vi "WriteBit.vi"(8 "Error In":errorcluster, 9 "State":bool, 10 "Line (1-14)":u8=1 min=1 max=14 step=1, 11 "Keithley 2602 In":refnum<visa-resource-name>) -> (0 "Error Out":errorcluster, 3 "Keithley 2602 Out":refnum<visa-resource-name>)   [LabVIEW 2012, in "Keithley-2602.lvlib"]
uses:
  Keithley-2602.lvlib
panel:
  out "concatenated string":string
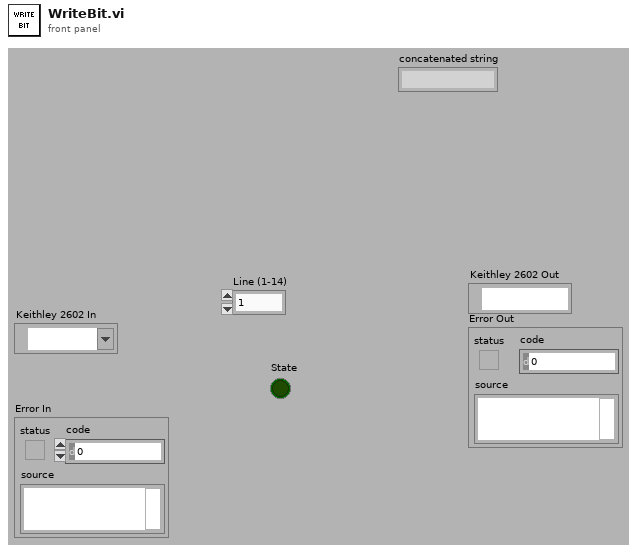
[diagram p1: front panel]
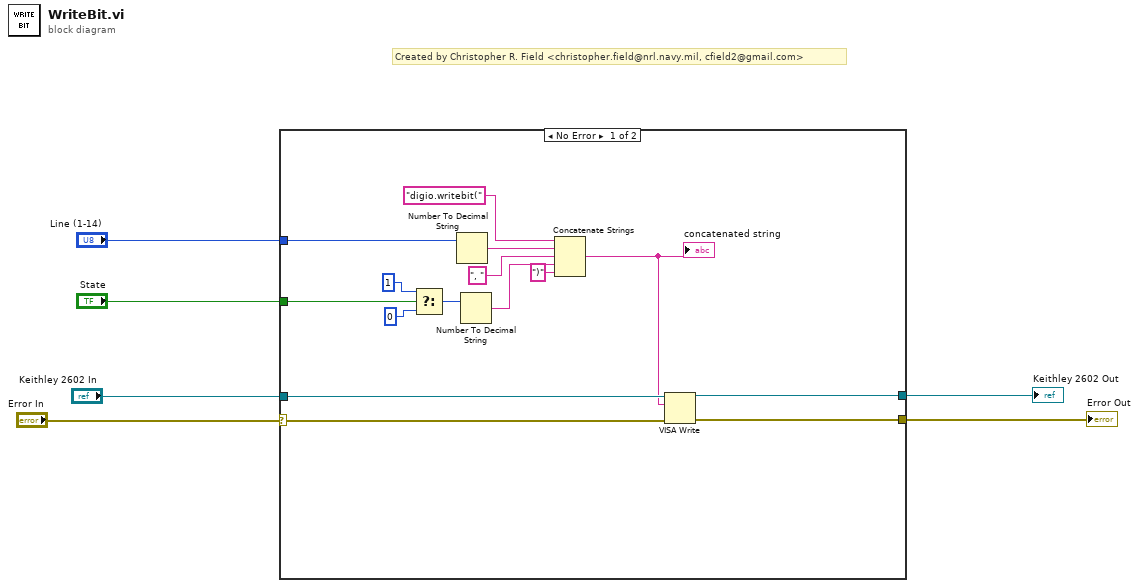
[diagram p0: block diagram]
diagram:
  # "Created by Christopher R. Field <christopher.field@nrl.navy.mil, cfield2@gmail.com>"
  n1 = case shown="No Error" "Error In" {
    selector: "Error In" -> [w7 w23]
    tunnel: "Keithley 2602 In" -> [w21 w22]
    tunnel: [w20 w22] -> w5
    tunnel: [w19 w23] -> w4
    tunnel: "Line (1-14)" -> [w18 _]
    tunnel: "State" -> [w13 _]
    frame No Error {
      n2 = Select(t=1, s=w13, f=0) -> (s? t:f=w10:i32)
      n3 = Number To Decimal String(number=w18) -> (decimal integer string=w16:string)  [unwired: 1 in]
      n4 = Number To Decimal String(number=w10) -> (decimal integer string=w9:string)  [unwired: 1 in]
      n5 = Concatenate Strings("digio.writebit(", w16, ", ", w9, ")" ("string")) -> (w14:string)
      "concatenated string" <- w14
      n6 = VISA Write(VISA resource name=w21, write buffer=w14, error in (no error)=w7) -> (VISA resource name out=w20:refnum<visa-resource-name>, error out=w19:errorcluster)  [unwired: 1 out]
    }
    frame Error {
    }
  }
  "Keithley 2602 Out" <- w5
  "Error Out" <- w4
